vi "Control Selection.vi"(3 "Only Enabled? (F)":bool, 4 "Controls In[]":refnum<vi>[](array[refnum]), 5 "Only Visible? (T)":bool=TRUE) -> (1 "Controls Out[]":refnum<vi>[](array[refnum]))   [LabVIEW 2009]
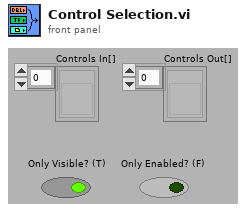
[diagram p1: front panel]
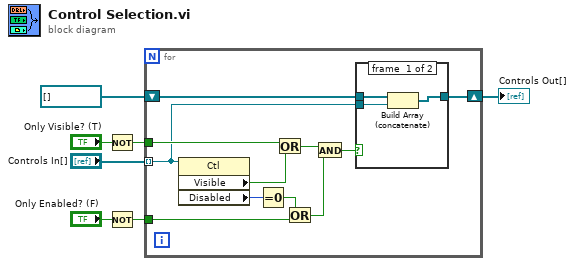
[diagram p0: block diagram]
diagram:
  n1 = Not(x="Only Visible? (T)") -> (.not. x?=w1:bool)
  n2 = Not(x="Only Enabled? (F)") -> (.not. x?=w2:bool)
  n3 = for {
    tunnel: "Controls In[]" -> [w9] mode=indexing
    tunnel: w1 -> [w17]
    tunnel: w2 -> [w15]
    shift-right: [w8] -> w7
    shift-left: refnum<vi>[] [] -> [w10]
    n4 = property class="Ctl"(reference=w9) -> ("Visible"=w16:bool, "Disabled"=w18:u8)  [unwired: 1 in, 2 out]
    n5 = Equal To 0?(x=w18) -> (x = 0?=w14:bool)
    n6 = Or(x=w17, y=w16) -> (x .or. y?=w13:bool)
    n7 = Or(x=w14, y=w15) -> (x .or. y?=w12:bool)
    n8 = And(x=w13, y=w12) -> (x .and. y?=w11:bool)
    n9 = case shown="True" w11 {
      tunnel: w10 -> [w21 w22]
      tunnel: w9 -> [w20 _]
      tunnel: [w19 w22] -> w8
      frame #0 {
        n10 = Build Array (concatenate)(w21, w20) -> (w19:refnum<vi>[])
      }
      frame #1 {
      }
    }
  }
  "Controls Out[]" <- w7
